vi "Annotate Image and Save.vi"(7 "Mode":string, 8 "error in (no error)":errorcluster, 10 "Fiducial Image Positions":refnum<class "Vec3d.lvclass">[](array[class]), 11 "Fiducial Image":T2) -> (0 "error out":errorcluster, 3 "Fiducial Image out":T2)   [LabVIEW 2024]
uses:
  Vec3d Class/Vec3d.lvclass
  Vision/Vision.lvlib
  <vilib>/vision/Image Controls.llb/IMAQ Image.ctl
  Type Definitions/Physical Image.ctl
panel:
  out "Image":T1(plugin-control)
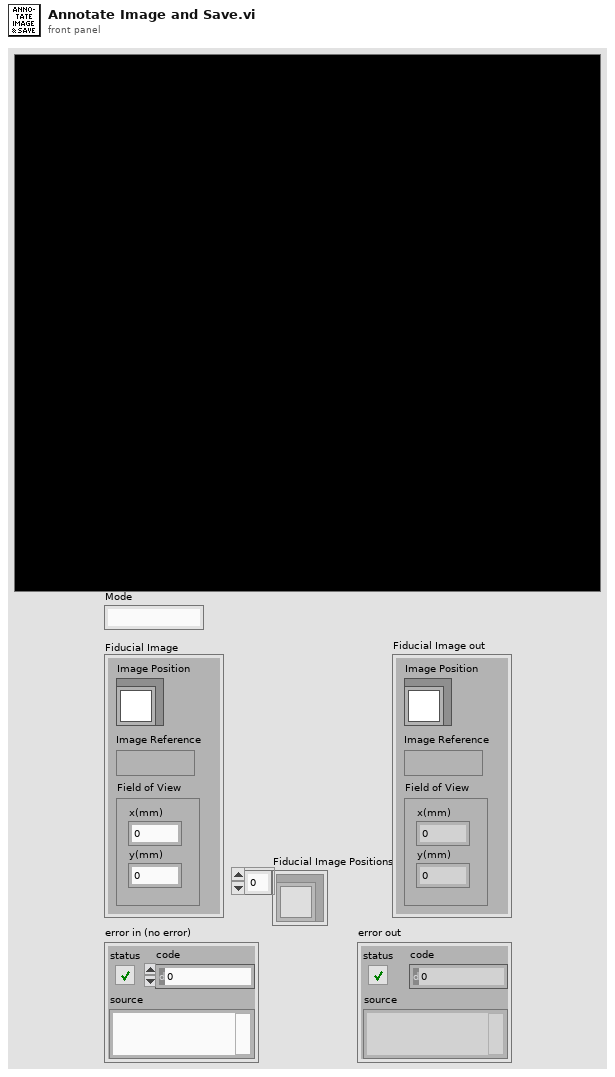
[diagram p1: front panel]
types:
  T1 = typedef "IMAQ Image.ctl" = refnum<image>
  T2 = typedef "Physical Image.ctl" = cluster{"Image Position":refnum<class "Vec3d.lvclass">, "Image Reference":T1, "Field of View":cluster{"x(mm)":dbl, "y(mm)":dbl}}
  T3 = enum32{"Invalid", "Standard", "Closed", "Hidden", "Minimized", "Maximized"}
  T4 = cluster{"Left":i32, "Top":i32, "Right":i32, "Bottom":i32}
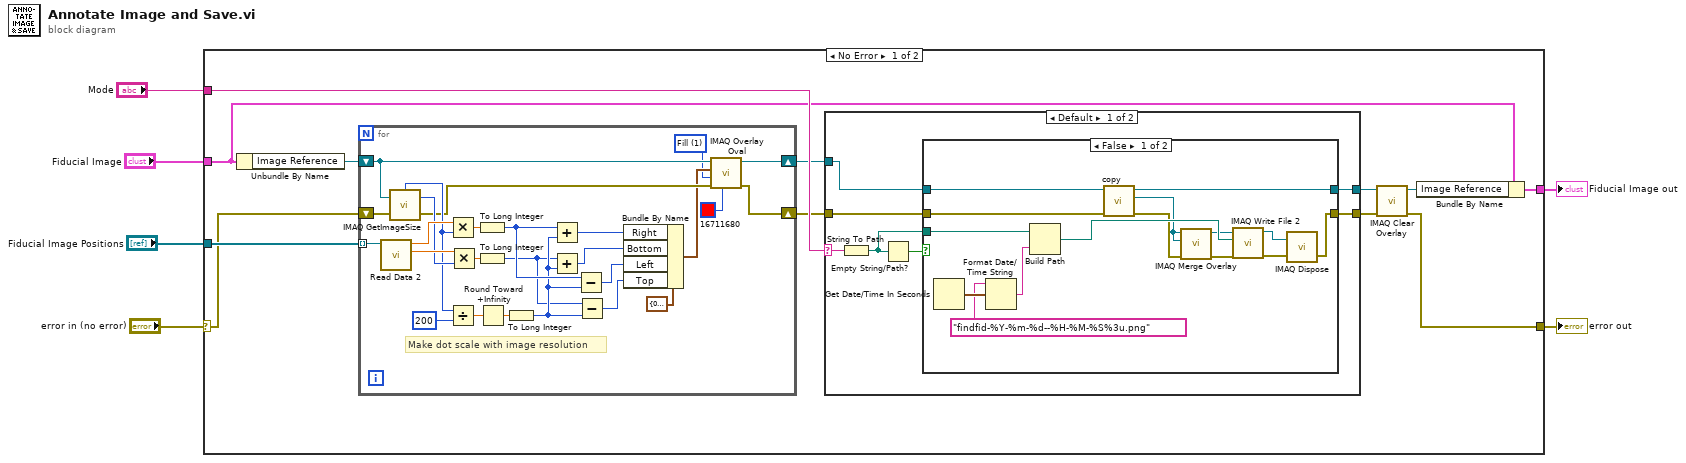
[diagram p0: block diagram]
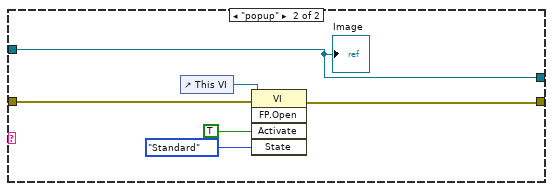
[diagram p3: hidden frame]
diagram:
  n1 = case shown="No Error" "error in (no error)" {
    selector: "error in (no error)" -> [w16 w76]
    tunnel: [w10 w76] -> w5
    tunnel: "Fiducial Image" -> [w9 w75]
    tunnel: "Fiducial Image Positions" -> [w18 _]
    tunnel: "Mode" -> [w15 _]
    tunnel: [w7 w75] -> w1
    frame No Error {
      n2 = Unbundle By Name(w9) -> ("Image Reference"=w17:T1)
      n3 = for {
        tunnel: w18 -> [w74] mode=indexing
        shift-right: [w52] -> w14
        shift-left: w17 -> [w68]
        shift-right: [w53] -> w13
        shift-left: w16 -> [w55]
        w50 = u32 1 items=["Frame", "Fill"] ("Drawing Mode (Frame)")
        # "Make dot scale with image resolution"
        n4 = call-dynamic "Read Data 2.vi"("Vec3d in"=w74) -> ("Y"=w72:dbl, "X"=w73:dbl)  [unwired: 7 in, 2 out]
        n5 = call "IMAQ GetImageSize"("Image"=w68, "error in (no error)"=w55) -> ("Y Resolution"=w71:i32, "X Resolution"=w67:i32, "error out"=w54:errorcluster)  [unwired: 2 in]
        n6 = Multiply(x=w73, y=w67) -> (x*y=w70:dbl)
        n7 = Divide(x=w67, y=200) -> (x/y=w65:dbl)
        n8 = Multiply(x=w72, y=w71) -> (x*y=w69:dbl)
        n9 = To Long Integer(number=w70) -> (32bit integer=w63:i32)
        n10 = To Long Integer(number=w69) -> (32bit integer=w61:i32)
        n11 = Round Toward +Infinity(x=w65) -> (ceil(x): smallest int >= x=w64:dbl)
        n12 = To Long Integer(number=w64) -> (32bit integer=w62:i32)
        n13 = Add(x=w63, y=w62) -> (x+y=w59:i32)
        n14 = Add(x=w61, y=w62) -> (x+y=w58:i32)
        n15 = Subtract(x=w63, y=w62) -> (x-y=w57:i32)
        n16 = Subtract(x=w61, y=w62) -> (x-y=w56:i32)
        n17 = Bundle By Name(cluster=T4 {"Left"=0, "Top"=0, "Right"=0, "Bottom"=0} ("Bounding Rectangle"), "Right"=w59, "Bottom"=w58, "Left"=w57, "Top"=w56) -> (w51:T4)
        n18 = call "IMAQ Overlay Oval"("Color"=u32 16711680, "error in (no error)"=w54, "Drawing Mode (Frame)"=w50, "Bounding Rectangle"=w51, "Image"=w68) -> ("error out"=w53:errorcluster, "Image Out"=w52:T1)  [unwired: 5 in]
      }
      n19 = case shown="Default" w15 {
        selector: w15 -> [w21 _]
        tunnel: w14 -> [w23 w48]
        tunnel: w13 -> [w25 w46]
        tunnel: [w22 w48] -> w12
        tunnel: [w24 w45] -> w11
        frame Default {
          n20 = String To Path(string=w21) -> (path=w20:path)
          n21 = Empty String/Path?(string/path=w20) -> (empty?=w19:bool)
          n22 = case shown="False" w19 {
            tunnel: w25 -> [w29 w42]
            tunnel: [w34 w42] -> w24
            tunnel: w23 -> [w30 w41]
            tunnel: [w28 w41] -> w22
            tunnel: w20 -> [w38 _]
            frame False {
              n23 = Get Date/Time In Seconds() -> (seconds since 1Jan1904=w40:timestamp)
              n24 = Format Date/Time String(time format string (%c)="findfid-%Y-%m-%d--%H-%M-%S%3u.png", seconds (now)=w40) -> (date/time string=w37:string)  [unwired: 1 in]
              n25 = Build Path(base path=w38, name or relative path=w37) -> (appended path=w33:path)
              n26 = call "copy.vi"("error in (no error)"=w29, "Image in"=w30) -> ("error out"=w26:errorcluster, "copy"=w27:T1, "original"=w28:T1)  [unwired: 5 in]
              n27 = call "IMAQ Merge Overlay"("error in (no error)"=w26, "Image Dst"=w27, "Image Src"=w27) -> ("error out"=w31:errorcluster, "Image Dst Out"=w32:T1)  [unwired: 7 in]
              n28 = call-poly "IMAQ Write File 2"("error in (no error)"=w31, "File Path"=w33, "Image"=w32) -> ("error out"=w35:errorcluster, "Image Out (duplicate)"=w36:T1)  [unwired: 7 in]
              n29 = call "IMAQ Dispose"("Image"=w36, "error in (no error)"=w35) -> ("error out"=w34:errorcluster)  [unwired: 4 in]
            }
            frame True {
            }
          }
        }
        frame "popup" {
          n30 = control-ref of="This VI"() -> (w47:refnum<vi>)
          n31 = invoke class="VI" method="FP.Open"(reference=w47, error in=w46, "Activate"=TRUE ("Activate?"), "State"=T3."Standard") -> (error out=w45:errorcluster)  [unwired: 1 in, 4 out]
          "Image" <- w48
        }
      }
      n32 = call "IMAQ Clear Overlay"("error in (no error)"=w11, "Image"=w12) -> ("error out"=w10:errorcluster, "Image Out"=w8:T1)  [unwired: 8 in]
      n33 = Bundle By Name(cluster=w9, "Image Reference"=w8) -> (w7:T2)
    }
    frame Error {
    }
  }
  "error out" <- w5
  "Fiducial Image out" <- w1
